vi "test_RemoteScopeSession_CallCloseMeasurementLinkSessionWithCloseBehavior_RemoteSessionClosed.vi"(8 "error in":errorcluster) -> (0 "error out":errorcluster, 2 "result":string, 3 "pass":bool)   [LabVIEW 2020, in "MeasurementServerTests.lvlib"]
uses:
  MeasurementServerTests.lvlib
  Runtime/MeasurementLink Instrument/IInstrument/Close Session Behavior.ctl
  Runtime/MeasurementLink Instrument/IInstrument/IInstrument.lvclass
  Runtime/MeasurementLink niScope/Instrument/Instrument.lvclass
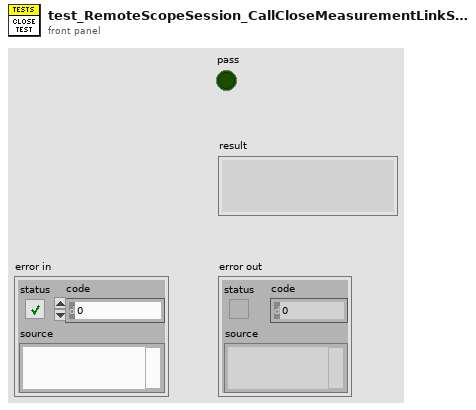
[diagram p1: front panel]
types:
  T1 = typedef "MeasurementLink Instrument.lvlib/IInstrument.lvclass/Remote Connection Options.ctl" = cluster{"session name":string, "address":string, "port":u32}
  T2 = typedef "MeasurementLink Instrument.lvlib/IInstrument.lvclass/Close Session Behavior.ctl" = enum16{"Close Session", "Detach Session"}
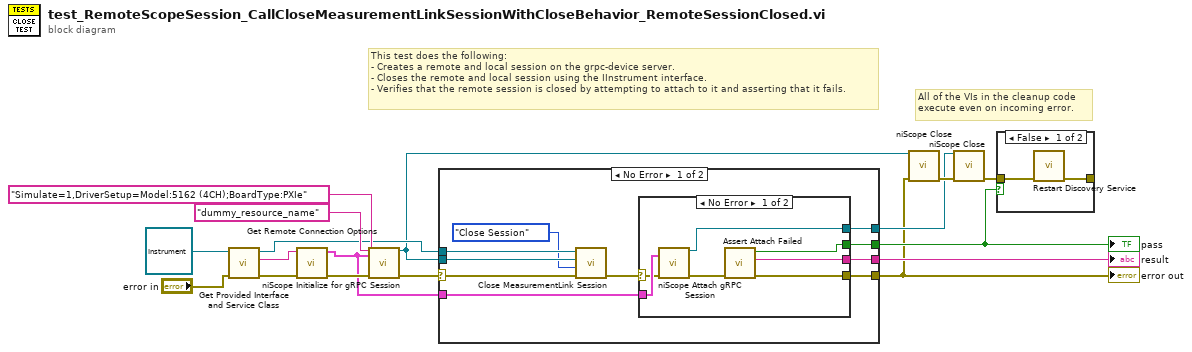
[diagram p0: block diagram]
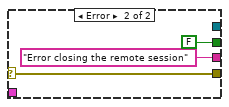
[diagram p2: hidden frame]
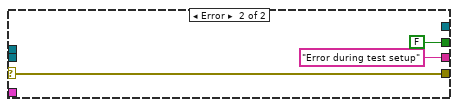
[diagram p3: hidden frame]
diagram:
  # "All of the VIs in the cleanup code\nexecute even on incoming error."
  # "This test does the following:\n- Creates a remote and local session on the grpc-device server.\n- Closes the remote and local session using the IInstrument interface.\n- Verifies that the remote session is closed by attempting to attach to it and asserting that it fails."
  n1 = call-dynamic "Get Provided Interface and Service Class.vi"("error in"="error in", "instrument in"=refnum<class "Instrument.lvclass"> refnum ("MeasurementLink niScope.lvlib:Instrument.lvclass")) -> ("error out"=w14:errorcluster, "provided interface"=w13:string, "instrument out"=w10:refnum<class "Instrument.lvclass">)  [unwired: 6 in, 1 out]
  n2 = call "Get Remote Connection Options.vi"("error in"=w14, "provided interface"=w13) -> ("error out"=w16:errorcluster, "remote connection options"=w9:T1)  [unwired: 8 in]
  n3 = call <instrlib>:"niScope Initialize for gRPC Session.vi"("resource name"="dummy_resource_name", "gRPC options"=w9, "option string"="Simulate=1,DriverSetup=Model:5162 (4CH);BoardType:PXIe", "error in"=w16) -> ("instrument handle"=w5:refnum<k15>, "error out"=w11:errorcluster)  [unwired: 10 in]
  n4 = case shown="No Error" w11 {
    selector: w11 -> [w27 w39]
    tunnel: w10 -> [w26 _]
    tunnel: w5 -> [w25 _]
    tunnel: w9 -> [w24 _]
    tunnel: [w22 w39] -> w1
    tunnel: [w21 FALSE] -> w6
    tunnel: [w20 "Error during test setup" ("f")] -> w7
    tunnel: [w18 _] -> w3
    frame No Error {
      n5 = call-dynamic "Close MeasurementLink Session.vi"("error in"=w27, "close session behavior"=Close_Session_Behavior."Close Session", "session in"=w25, "instrument in"=w26) -> ("error out"=w23:errorcluster)  [unwired: 7 in]
      n6 = case shown="No Error" w23 {
        selector: w23 -> [w33 w35]
        tunnel: w24 -> [w34 _]
        tunnel: [w30 w35] -> w22
        tunnel: [w32 FALSE] -> w21
        tunnel: [w29 "Error closing the remote session" ("f")] -> w20
        tunnel: [w28 _] -> w18
        frame No Error {
          n7 = call <instrlib>:"niScope Attach gRPC Session.vi"("gRPC options"=w34, "error in"=w33) -> ("instrument handle"=w28:refnum<k15>, "error out"=w31:errorcluster)  [unwired: 12 in]
          n8 = call "Assert Attach Failed.vi"("error in"=w31) -> ("error out"=w30:errorcluster, "result"=w29:string, "pass?"=w32:bool)  [unwired: 8 in]
        }
        frame Error {
        }
      }
    }
    frame Error {
    }
  }
  "error out" <- w1
  "pass" <- w6
  "result" <- w7
  n9 = call <instrlib>:"niScope Close.vi"("instrument handle"=w5, "error in"=w1) -> ("error out"=w4:errorcluster)  [unwired: 13 in]
  n10 = call <instrlib>:"niScope Close.vi"("instrument handle"=w3, "error in"=w4) -> ("error out"=w2:errorcluster)  [unwired: 13 in]
  n11 = case shown="False" w6 {
    tunnel: [w42 _] -> _
    tunnel: w2 -> [w41 _]
    frame False {
      n12 = call "Restart Discovery Service.vi"("error in"=w41) -> ("error out"=w42:errorcluster)  [unwired: 10 in]
    }
    frame True {
    }
  }
